vi "new imu.vi"(11 "error in (no error)":errorcluster) -> (0 "Numeric":dbl format="%#_13g", 3 "error out":errorcluster)   [LabVIEW 2015]
uses:
  <vilib>/myRIO/Instrument Drivers/Onboard IO/I2C/typedefs/I2C User Configuration.ctl
  <vilib>/myRIO/Instrument Drivers/Onboard IO/I2C/typedefs/I2C Transfer Rate.ctl
  <vilib>/myRIO/Instrument Drivers/Onboard IO/I2C/typedefs/I2C Reference.ctl
  <vilib>/myRIO/Common/Instrument Driver Framework/Utilities/typedefs/myRIO Generic Hardware Reference.ctl
  <vilib>/myRIO/Common/Instrument Driver Framework/Utilities/typedefs/Hardware Version Enum.ctl
  <vilib>/myRIO/Common/Instrument Driver Framework/Utilities/typedefs/myRIO v1.0 Reference.ctl
  <vilib>/myRIO/Common/Instrument Driver Framework/Utilities/typedefs/Generic FPGA Reference.ctl
  <vilib>/myRIO/Common/Instrument Driver Framework/myRIO v1.0/I2C/typedefs/I2C Channels Enum.ctl
  <vilib>/myRIO/Instrument Drivers/Onboard IO/I2C/typedefs/I2C Configuration.ctl
  <vilib>/userdefined/High Color/nirio_resource_hc.ctl
  <vilib>/myRIO/Common/Instrument Driver Framework/Utilities/vis/Is FPGA Ref Available.vi
  <vilib>/myRIO/Common/Instrument Driver Framework/myRIO v1.0/I2C/vis/myRIO v1.1 Open I2C.vi
  <vilib>/myRIO/Instrument Drivers/Onboard IO/I2C/vis/Configure.vi
  <vilib>/myRIO/Instrument Drivers/Onboard IO/I2C/vis/Write.vi
  <vilib>/myRIO/Instrument Drivers/Onboard IO/I2C/vis/Read.vi
  <vilib>/myRIO/Common/Instrument Driver Framework/Utilities/vis/Validate Channels.vi
  <vilib>/myRIO/Common/Instrument Driver Framework/myRIO v1.0/I2C/vis/myRIO v1.0 Reserve I2C.vi
  <vilib>/myRIO/Common/Instrument Driver Framework/myRIO v1.0/I2C/vis/myRIO v1.0 Build MUX Configuration I2C.vi
  <vilib>/myRIO/Common/Instrument Driver Framework/myRIO v1.0/Resource Manager/vis/myRIO v1.0 Reserve Channel List.vi
  <vilib>/myRIO/Common/Instrument Driver Framework/myRIO v1.0/Resource Manager/vis/myRIO v1.0 Create Configuration List.vi
  <vilib>/myRIO/Common/Instrument Driver Framework/myRIO v1.0/Resource Manager/vis/myRIO v1.0 Reserve Channel.vi
  <vilib>/myRIO/Common/Instrument Driver Framework/myRIO v1.0/Resource Manager/vis/myRIO v1.0 Unreserve Channel.vi
  <vilib>/myRIO/Common/Instrument Driver Framework/myRIO v1.0/Resource Manager/vis/myRIO v1.0 Build Mutex Name.vi
  <vilib>/Utility/VariantDataType/GetNumericInfo.vi
  <vilib>/Utility/error.llb/Error Cluster From Error Code.vi
  <vilib>/myRIO/Common/Instrument Driver Framework/myRIO v1.0/myRIO v1.1 Open.vi
  <vilib>/myRIO/Common/Instrument Driver Framework/Utilities/vis/IO Manager.vi
  <vilib>/myRIO/Common/Instrument Driver Framework/Utilities/vis/Configuration Manager.vi
  <vilib>/myRIO/Common/Instrument Driver Framework/myRIO v1.0/Resource Manager/vis/myRIO v1.0 Configure IO.vi
  <vilib>/myRIO/Common/Instrument Driver Framework/myRIO v1.0/myRIO v1.0 Close.vi
  <vilib>/myRIO/Common/Instrument Driver Framework/myRIO v1.0/I2C/vis/myRIO v1.0 Configure I2C.vi
  <vilib>/myRIO/Common/Instrument Driver Framework/myRIO v1.0/I2C/vis/myRIO v1.0 Write I2C.vi
  <vilib>/myRIO/Common/Instrument Driver Framework/myRIO v1.0/I2C/vis/myRIO v1.0 Read I2C.vi
  <vilib>/myRIO/Express VI/Onboard IO/I2C/I2C Express VI.xnode
  <vilib>/myRIO/Instrument Drivers/Onboard IO/I2C/vis/myRIO I2C Open.xnode
  <vilib>/myRIO/Instrument Drivers/Onboard IO/I2C/I2C.lvlib
panel:
  out "Heading Data":T1
  out "Array 2":u8[](array[numeric]) format="%b"
  out "Array":u8[](array[numeric]) format="%b"
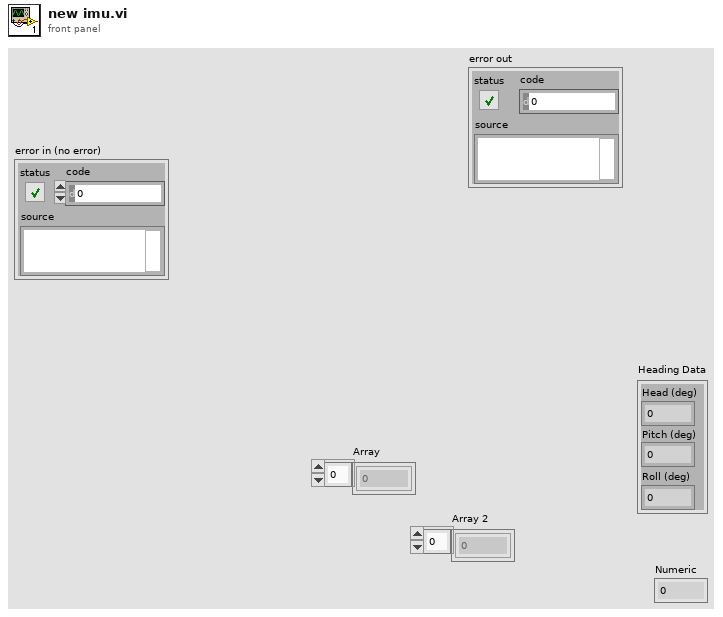
[diagram p1: front panel]
types:
  T1 = cluster{"Head (deg)":dbl, "Pitch (deg)":dbl, "Roll (deg)":dbl}
  T2 = typedef "I2C.lvlib/I2C Reference.ctl" = cluster{"myRIO Reference":T3, "I2C Channels Enum":T7, "I2C Configuration":T8}
  T3 = typedef "myRIO Generic Hardware Reference.ctl" = cluster{"myRIO Model":T4, "myRIO Hardware Reference":T5}
  T4 = typedef "Hardware Version Enum.ctl" = enum16{"Unknown", "myRIO-1900", "myRIO-1950", "roboRIO"}
  T5 = typedef "myRIO v1.0 Reference.ctl" = cluster{"Generic FPGA Reference":T6, "Allow multiple opens":bool}
  T6 = typedef "Generic FPGA Reference.ctl" = refnum<k20>
  T7 = typedef "I2C Channels Enum.ctl" = enum16{"Not Connected", "A/I2C", "B/I2C", "I2C/I2C"}
  T8 = typedef "I2C.lvlib/I2C Configuration.ctl" = cluster{"I2C Transfer Rate":T9}
  T9 = typedef "I2C.lvlib/I2C Transfer Rate.ctl" = enum16{"Standard mode (100 kbps)", "Fast mode (400 kbps)"}
  T10 = typedef "I2C.lvlib/I2C User Configuration.ctl" = cluster{"I2C Transfer Rate":T9}
  T11 = typedef "nirio_resource_hc.ctl" = tag
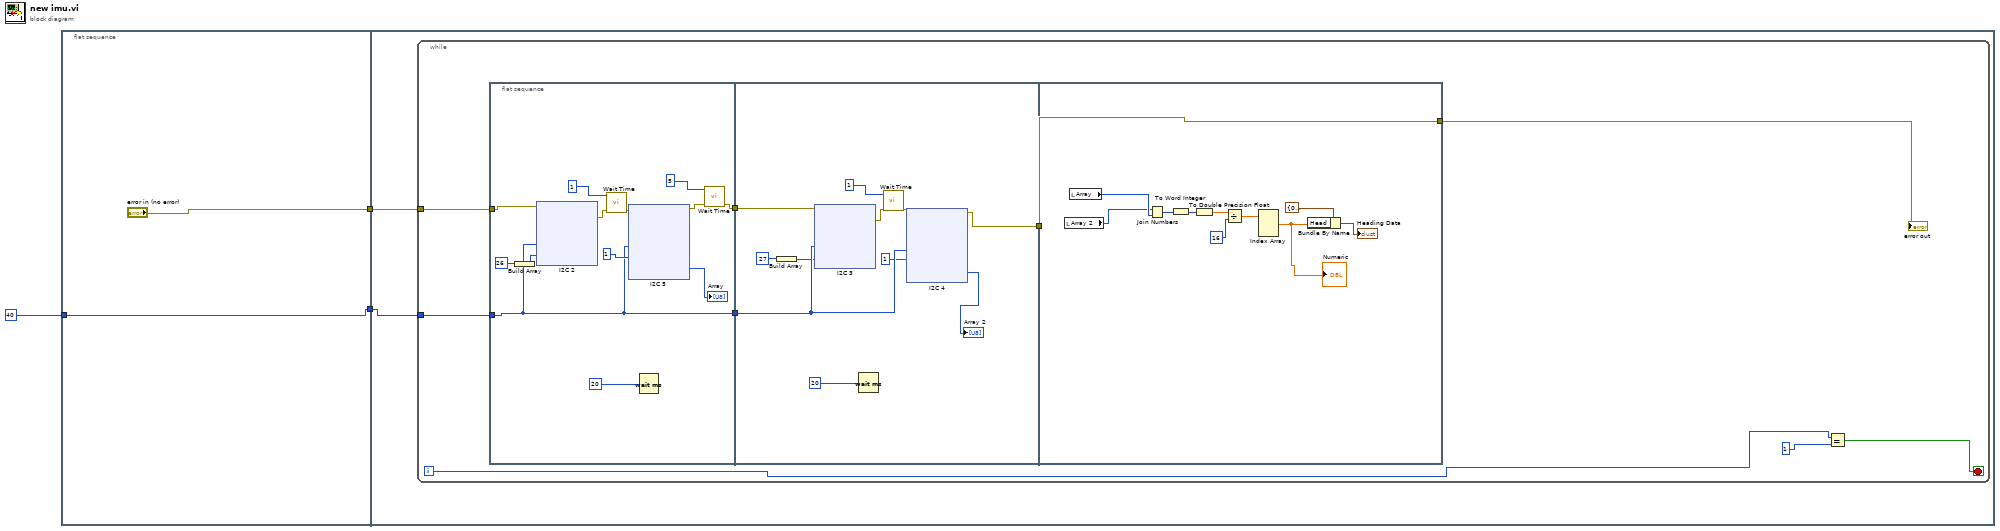
[diagram p0: block diagram]
diagram:
  n1 = flat-sequence {
    tunnel: ["error in (no error)"] -> w3
    tunnel: 40 -> [w5]
    tunnel: [w5] -> w1
    tunnel: w3 -> [w7]
    tunnel: w1 -> [w6]
    frame #0 {
    }
    frame #1 {
      n2 = while {
        tunnel: w7 -> [w12]
        tunnel: w6 -> [w11]
        i -> [w8]
        stop <- w10 stop-if-true
        n3 = flat-sequence {
          tunnel: [w19] -> w16
          tunnel: [w17] -> w15
          tunnel: w12 -> [w18]
          tunnel: w11 -> [w17]
          tunnel: w16 -> [w117]
          tunnel: [w116] -> w14
          tunnel: w15 -> [w115]
          tunnel: w14 -> [w205]
          tunnel: [w205] -> w13
          frame #0 {
            n4 = Build Array(26) -> (w26:i32[])
            n5 = xnode "I2C 2"("Slave Address (7-bit)"=w17, "Bytes to Write"=w26, "error in (no error)"=w18) -> ("error out"=w23:errorcluster)
            n6 = call "Wait Time.vi"("error in (no error)"=w23, "Wait Time (ms)"=1) -> ("error out"=w22:errorcluster)  [unwired: 9 in]
            n7 = xnode "I2C 5"("Slave Address (7-bit)"=w17, "Byte Count"=1, "error in (no error)"=w22) -> ("Bytes Read"=→"Array":u8[], "error out"=w20:errorcluster)
            n8 = Wait (ms)(milliseconds to wait=20) -> ()  [unwired: 1 out]
            n9 = call "Wait Time.vi"("error in (no error)"=w20, "Wait Time (ms)"=5) -> ("error out"=w19:errorcluster)  [unwired: 9 in]
          }
          frame #1 {
            n10 = Build Array(27) -> (w111:i32[])
            n11 = xnode "I2C 3"("Slave Address (7-bit)"=w115, "Bytes to Write"=w111, "error in (no error)"=w117) -> ("error out"=w108:errorcluster)
            n12 = Wait (ms)(milliseconds to wait=20) -> ()  [unwired: 1 out]
            n13 = call "Wait Time.vi"("error in (no error)"=w108, "Wait Time (ms)"=1) -> ("error out"=w107:errorcluster)  [unwired: 9 in]
            n14 = xnode "I2C 4"("Slave Address (7-bit)"=w115, "Byte Count"=1, "error in (no error)"=w107) -> ("Bytes Read"=→"Array 2":u8[], "error out"=w116:errorcluster)
          }
          frame #2 {
            n15 = local read "Array 2"() -> (w195:u8[])
            n16 = local read "Array"() -> (w196:u8[])
            n17 = Join Numbers(hi=w195, lo=w196) -> ((hi.lo)=w202:u16[])
            n18 = To Word Integer(number=w202) -> (16bit integer=w201:i16[])
            n19 = To Double Precision Float(number=w201) -> (double precision float=w200:dbl[])
            n20 = Divide(x=w200, y=16) -> (x/y=w199:dbl[])
            n21 = Index Array(array=w199) -> (element #1=w197:dbl)  [unwired: 3 in, 2 out]
            "Numeric" <- w197
            n22 = Bundle By Name(cluster=cluster{"Head":dbl, "Pitch":dbl, "Roll":dbl} {"Head"=0.0, "Pitch"=0.0, "Roll"=0.0} ("Heading Data"), "Head"=w197) -> (→"Heading Data":cluster{"Head":dbl, "Pitch":dbl, "Roll":dbl})
          }
        }
        n23 = Equal?(x=w8, y=1) -> (x = y?=w10:bool)
        "error out" <- w13
      }
    }
  }
